vi "Configure Interval.vi"(0 "VISA resource name":refnum<visa-resource-name>, 5 "Measurement Group (1)":i32=1 min=1 max=2, 7 "Scan Interval (0: 100ms)":u16(ring) items=["100ms", "200ms", "500ms", "1s", "2s", "5s", "1ms", "2ms", "5ms", "10ms", "20ms", "50ms"], 11 "error in (no error)":errorcluster) -> (4 "VISA resource name out":refnum<visa-resource-name>, 6 "Measurement Group":i32, 15 "error out":errorcluster)   [LabVIEW 2020, in "Yokogawa GX Series.lvlib"]
doc: "Sets the scan interval.\n\nCommand: SScan."
uses:
  <instrlib>/Yokogawa GX Series/Yokogawa GX Series.lvlib
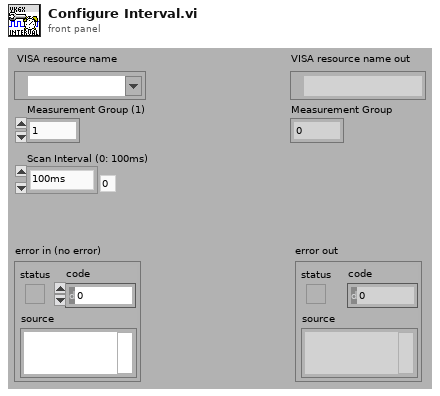
[diagram p1: front panel]
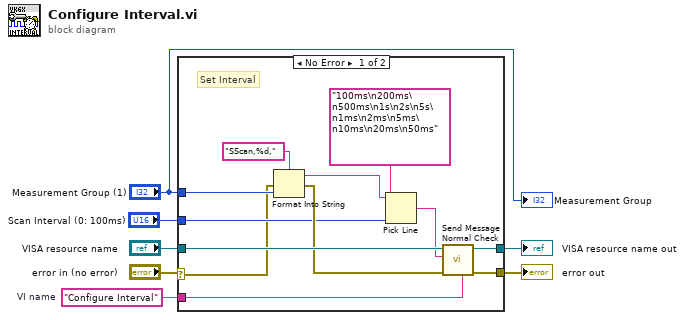
[diagram p0: block diagram]
diagram:
  w1 = "Configure Interval"  # VI name
  n1 = case shown="No Error" "error in (no error)" {
    selector: "error in (no error)" -> [w9 w20]
    tunnel: [w19 w21] -> w7
    tunnel: [w18 w20] -> w6
    tunnel: "VISA resource name" -> [w17 w21]
    tunnel: "Scan Interval (0: 100ms)" -> [w14 _]
    tunnel: "Measurement Group (1)" -> [w10 _]
    tunnel: w1 -> [w8 _]
    frame No Error {
      # "Set Interval"
      n2 = Format Into String(format string="SScan,%d,", error in=w9, w10) -> (resulting string=w12:string, error out=w15:errorcluster)  [unwired: 1 in]
      n3 = Pick Line(string ("")=w12, multi-line string="100ms\n200ms\n500ms\n1s\n2s\n5s\n1ms\n2ms\n5ms\n10ms\n20ms\n50ms", line index=w14) -> (output string=w13:string)
      n4 = call <instrlib>:"Send Message Normal Check.vi"("Source (\"\")"=w8, "error in (no error)"=w15, "Send Message (\"\")"=w13, "VISA resource name"=w17) -> ("error out"=w18:errorcluster, "VISA resource name out"=w19:refnum<visa-resource-name>)  [unwired: 2 in, 4 out]
    }
    frame Error {
    }
  }
  "error out" <- w6
  "VISA resource name out" <- w7
  "Measurement Group" <- "Measurement Group (1)"
